vi "AlGaAs_seq_v00.vi"(2 "Debug Mode":bool, 3 "Elapsed Time(s)":dbl, 4 "State":enum16{"Edit", "Start", "Run", "End", "Idle"}(ring), 5 "Argument List In":string[](array[string])) -> (0 "Status Out":string, 1 "Argument List Out":string[](array[string]))   [LabVIEW 2011]
panel:
  out "time array":dbl[](array[numeric])
  out "nPeriod":dbl
  out "tTotal(s) 2":dbl
  out "is_OK":bool
  out "tSequence(s)":dbl
  in  "Tab Control":enum32{"Step 1", "Step 2", "Step 3", "Step 4"}(tab)
  in  "run Ga 1":bool caption="run Ga"
  in  "run Al 1":bool caption="run Al"
  in  "Al flow 1":dbl caption="Al flow(0-100sccm)" format="%.1f"
  in  "time 1":dbl caption="time(s)"
  in  "Ga flow 1":dbl caption="Ga flow(0-10sccm)" format="%.3f"
  in  "fGa dilution 1":dbl=1.0 caption="fGa dilution(>=1)"
  in  "run Ga 2":bool caption="run Ga"
  in  "run Al 2":bool caption="run Al"
  in  "fGa dilution 2":dbl=1.0 caption="fGa dilution(>=1)"
  in  "Al flow 2":dbl caption="Al flow (0-100sccm)" format="%.1f"
  in  "Ga flow 2":dbl caption="Ga flow (0-10sccm)" format="%.3f"
  in  "time 2":dbl caption="time(s)"
  in  "time 3":dbl caption="time(s)"
  in  "Al flow 3":dbl caption="Al flow (0-100sccm)" format="%.1f"
  in  "run Al 3":bool caption="run Al"
  in  "Ga flow 3":dbl caption="Ga flow (0-10sccm)" format="%.3f"
  in  "fGa dilution 3":dbl=1.0 caption="fGa dilution(>=1)"
  in  "run Ga 3":bool caption="run Ga"
  in  "time 4":dbl caption="time(s)"
  in  "Al flow 4":dbl caption="Al flow (0-100sccm)" format="%.1f"
  in  "run Al 4":bool caption="run Al"
  in  "Ga flow 4":dbl caption="Ga flow (0-10sccm)" format="%.3f"
  in  "fGa dilution 4":dbl=1.0 caption="fGa dilution(>=1)"
  in  "run Ga 4":bool caption="run Ga"
  out "tphase(s)":dbl[](array[numeric])
  out "phase":i32
  in  "Cancel":bool
  in  "OK":bool
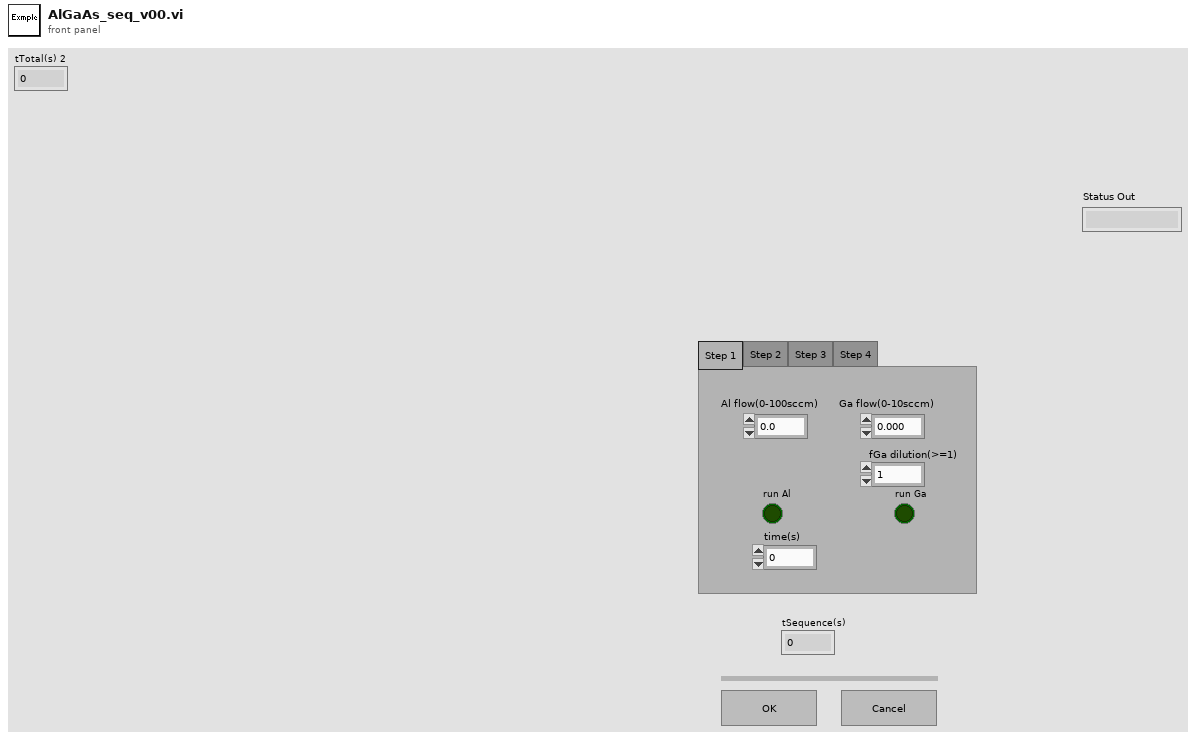
[diagram p1: front panel]
types:
  T1 = enum16{"Discrete", "Continuous", "Instantaneous"}
  T2 = enum32{"Invalid", "Default", "Floating", "Floating/Auto-Hide", "Modal"}
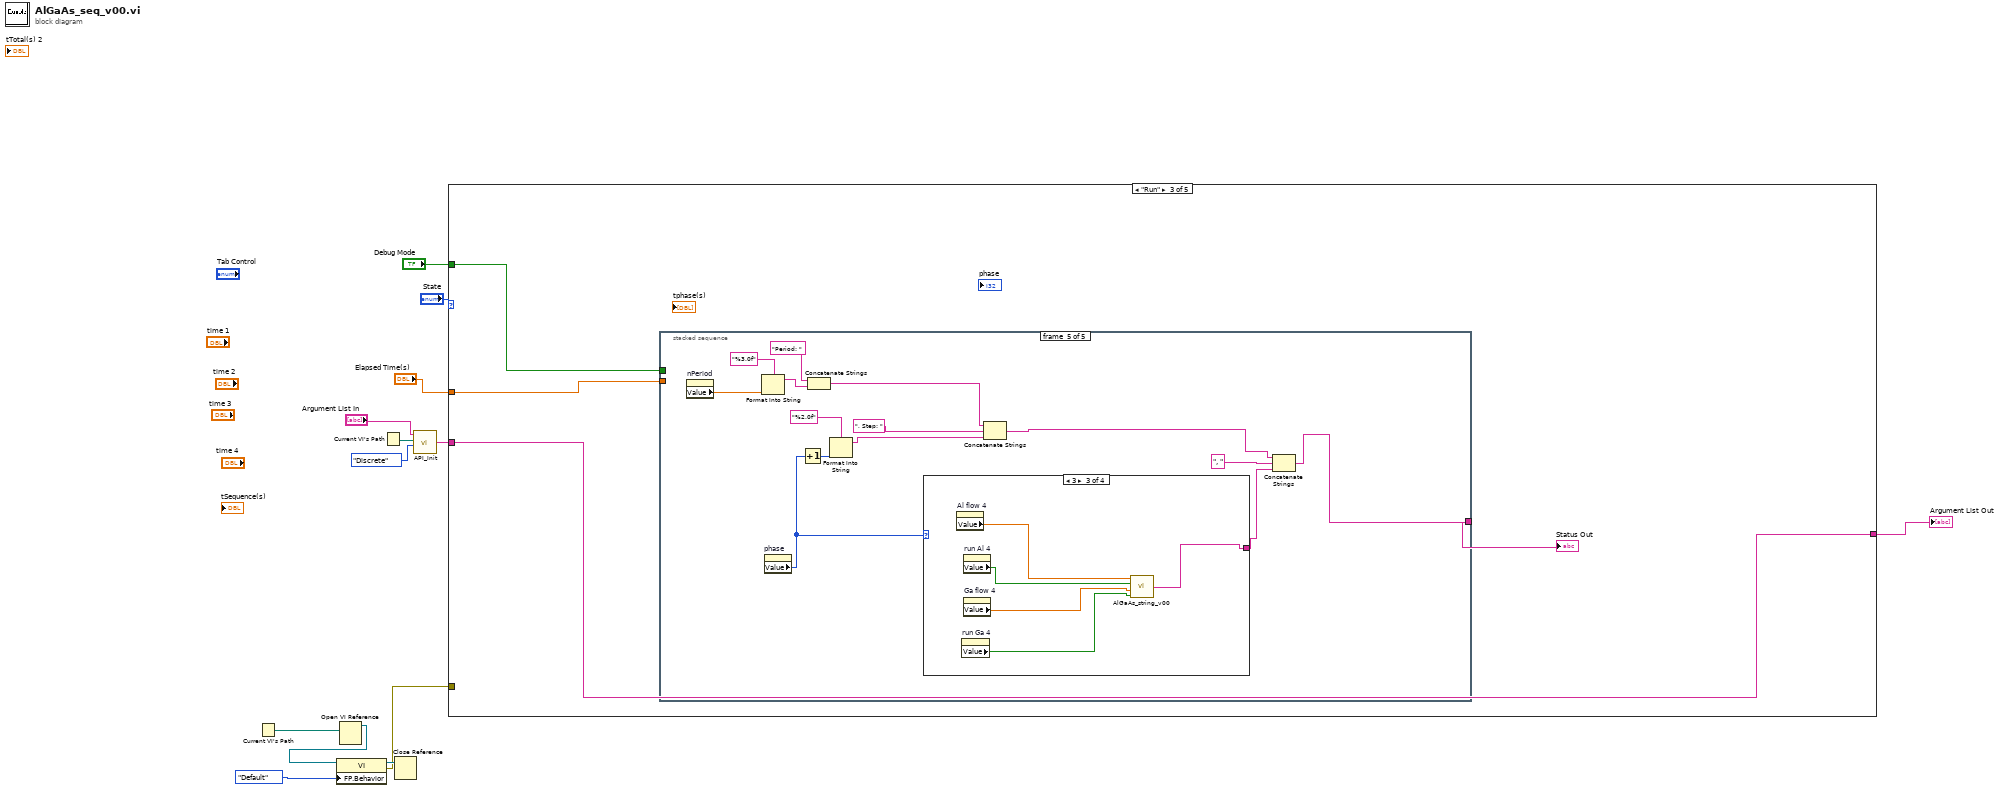
[diagram p0: block diagram]
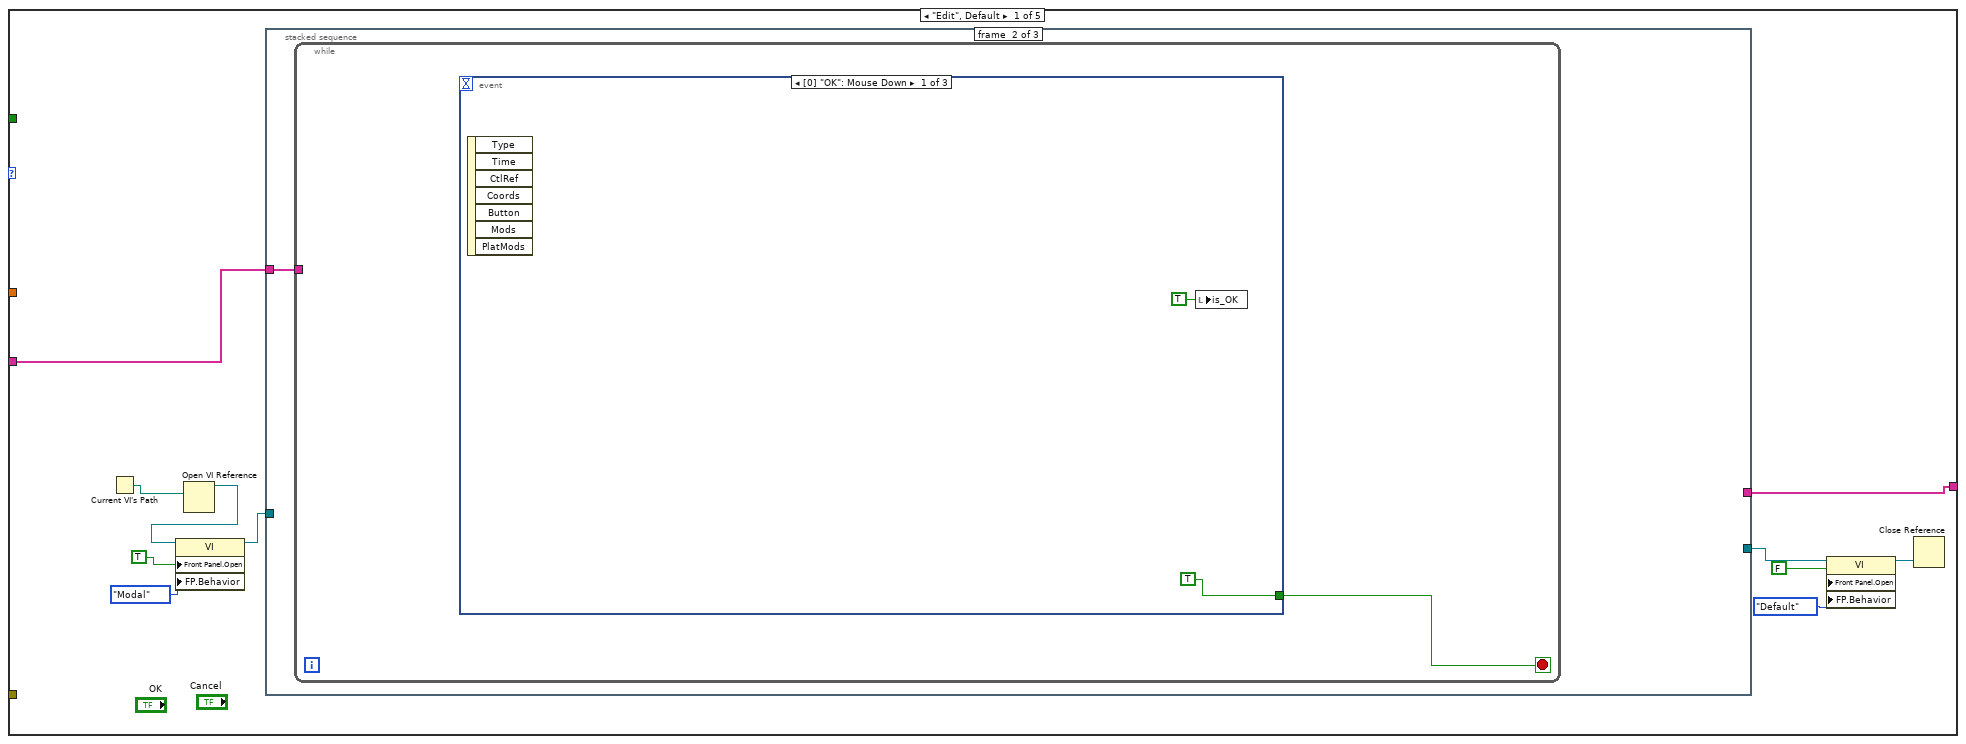
[diagram p2: hidden frame]
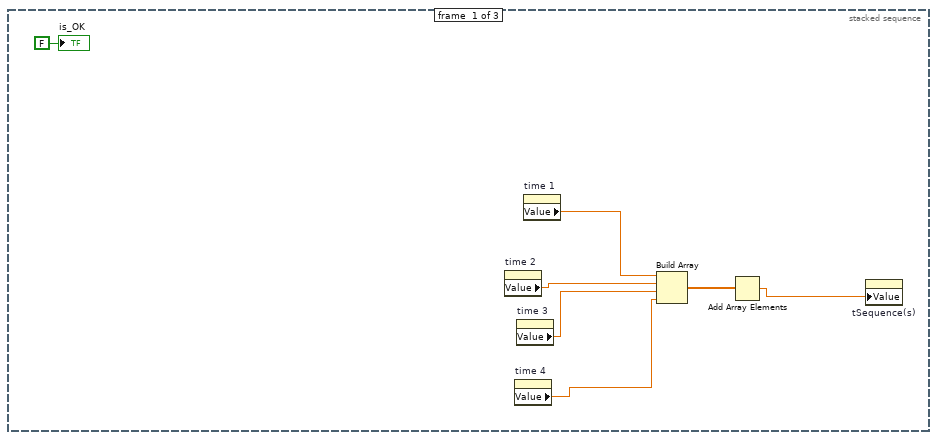
[diagram p3: hidden frame]
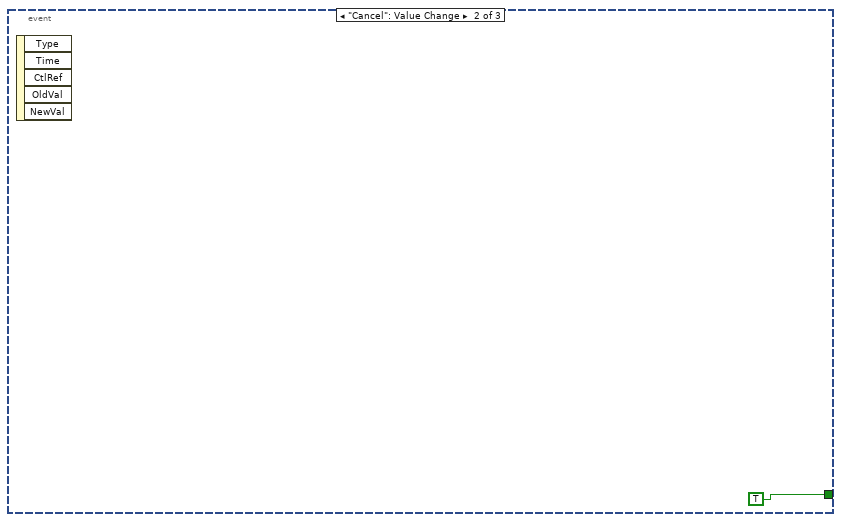
[diagram p4: hidden frame]
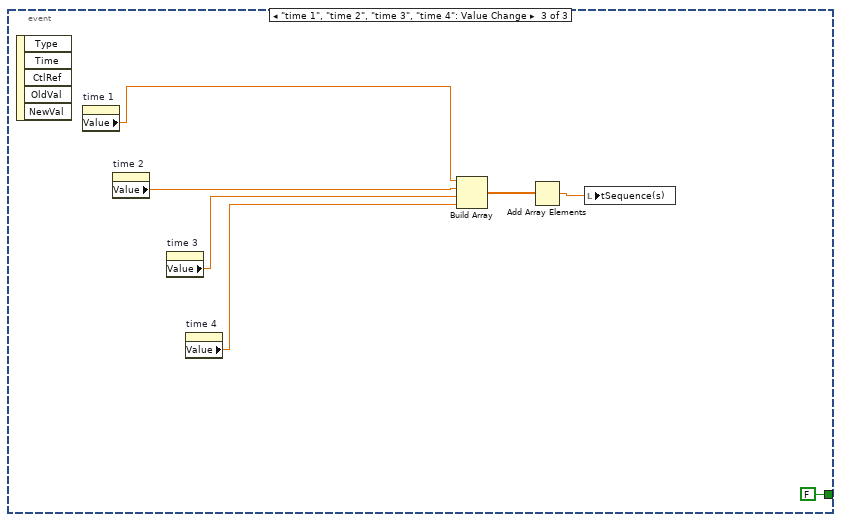
[diagram p5: hidden frame]
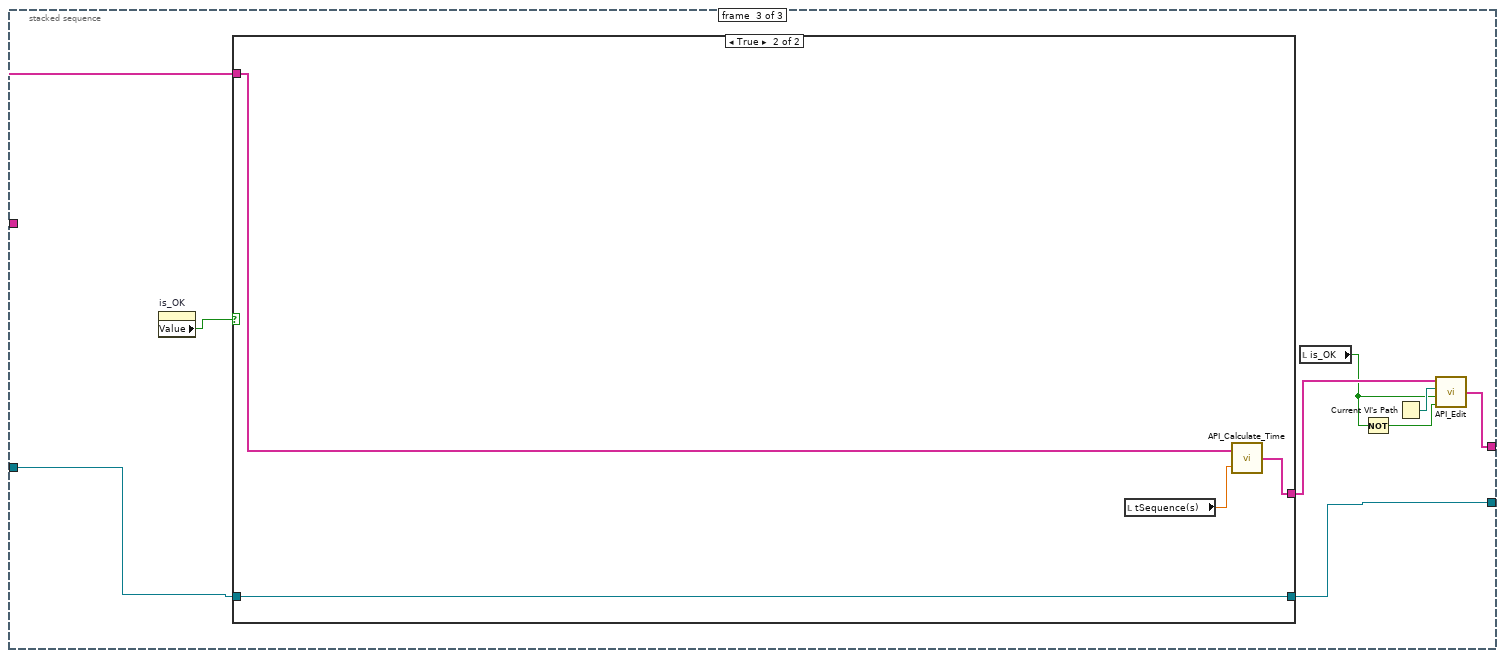
[diagram p6: hidden frame]
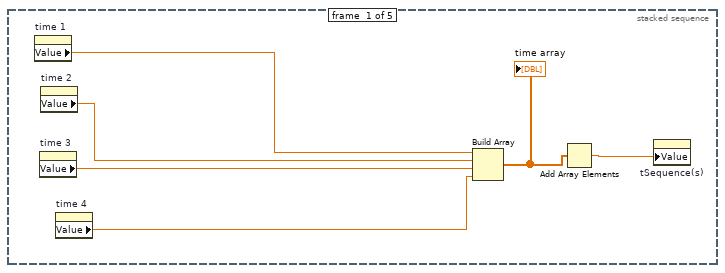
[diagram p9: hidden frame]
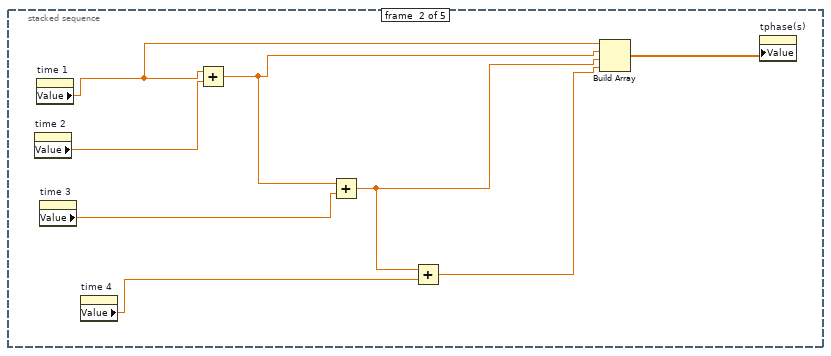
[diagram p10: hidden frame]
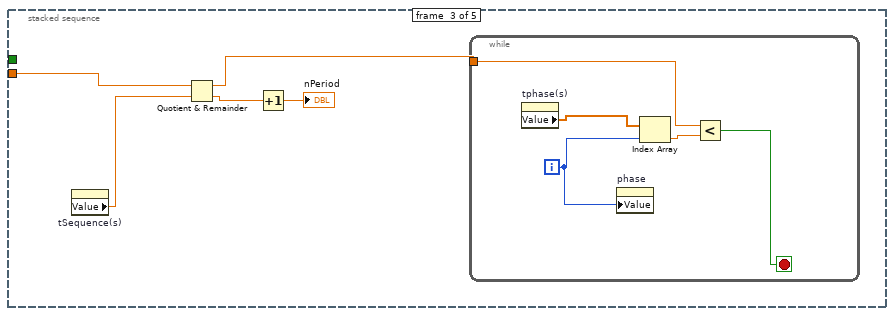
[diagram p11: hidden frame]
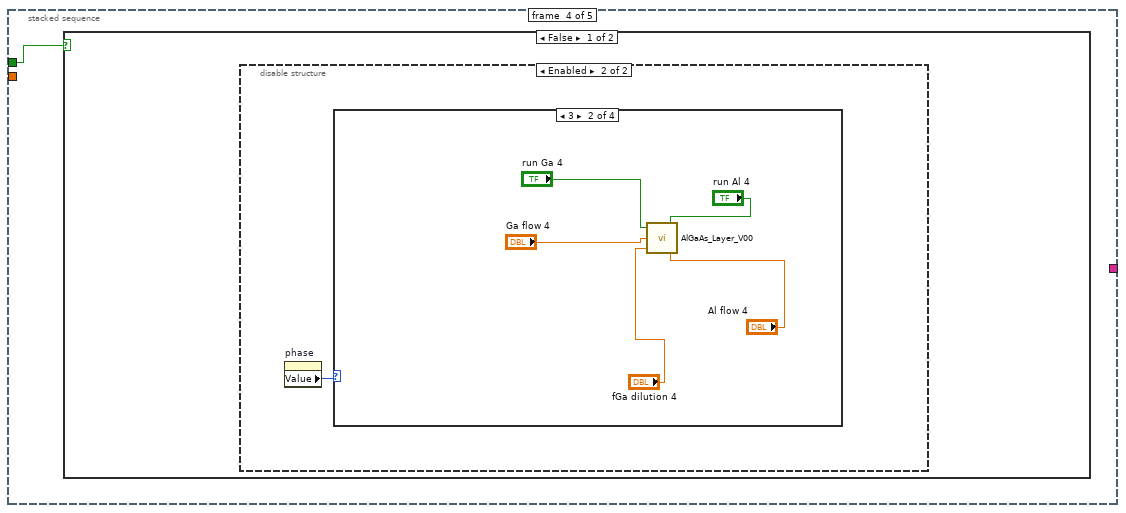
[diagram p12: hidden frame]
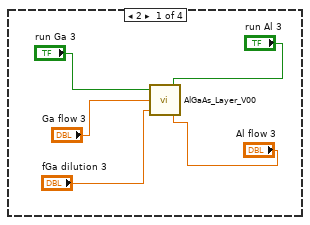
[diagram p14: hidden frame]
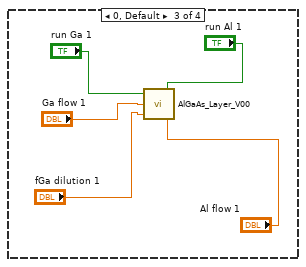
[diagram p15: hidden frame]
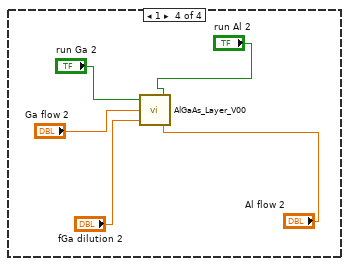
[diagram p16: hidden frame]
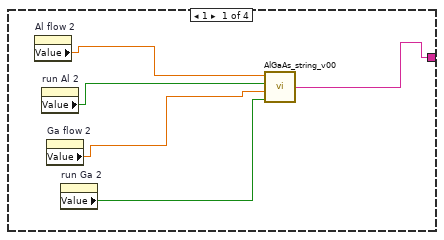
[diagram p18: hidden frame]
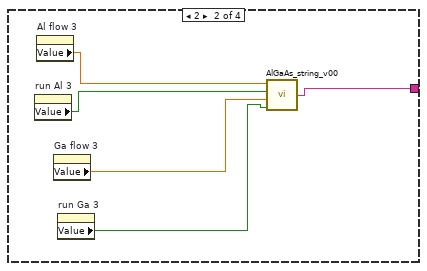
[diagram p19: hidden frame]
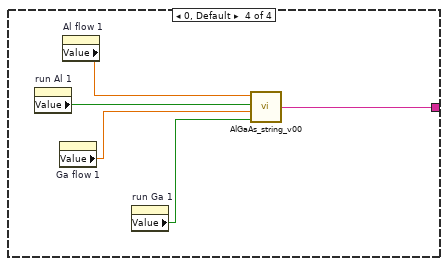
[diagram p20: hidden frame]
diagram:
  n1 = Current VI's Path() -> (path=w9:path)
  n2 = Open VI Reference(vi path=w9) -> (vi reference=w8:refnum<vi>)  [unwired: 1 in, 5 out]
  n3 = property class="VI"(reference=w8, "FP.Behavior"=T2."Default" ("Front Panel Window:Behavior")) -> (reference out=w6:refnum<vi>, error out=w5:errorcluster)  [unwired: 1 in]
  n4 = Current VI's Path() -> (path=w4:path)
  n5 = Close Reference(reference=w6) -> ()  [unwired: 1 in, 1 out]
  n6 = call "API_Init.vi"("API Mode"=T1."Discrete", "VI Path"=w4, "Argument List In"="Argument List In") -> ("Argument List Out"=w1:string[])  [unwired: 1 in]
  n7 = case shown="\"Run\"" "State" {
    tunnel: "Debug Mode" -> [_ _ w62 _ _]
    tunnel: "Elapsed Time(s)" -> [_ _ w63 _ _]
    tunnel: w1 -> [w14 w59 w60 w144 w145]
    tunnel: [w21 w59 w60 w144 w145] -> w10
    tunnel: w5 -> [_ _ _ _ _]
    frame "Edit", Default {
      n8 = Current VI's Path() -> (path=w19:path)
      n9 = Open VI Reference(vi path=w19) -> (vi reference=w18:refnum<vi>)  [unwired: 1 in, 5 out]
      n10 = property class="VI"(reference=w18, "Front Panel.Open"=TRUE ("Front Panel Window:Open"), "FP.Behavior"=T2."Modal" ("Front Panel Window:Behavior")) -> (reference out=w17:refnum<vi>)  [unwired: 1 in, 1 out]
      n11 = stacked-sequence {
        tunnel: w14 -> [_ w32 w52]
        tunnel: w17 -> [_ _ w50]
        tunnel: [_ _ w49] -> w22
        tunnel: [_ _ w46] -> w21
        frame #0 {
          n12 = property on="time 2" class="DigNum (strict)"() -> ("Value"=w27:dbl)  [unwired: 2 in, 2 out]
          n13 = property on="time 4" class="DigNum (strict)"() -> ("Value"=w25:dbl)  [unwired: 2 in, 2 out]
          n14 = property on="time 3" class="DigNum (strict)"() -> ("Value"=w26:dbl)  [unwired: 2 in, 2 out]
          n15 = property on="time 1" class="DigNum (strict)"() -> ("Value"=w30:dbl)  [unwired: 2 in, 2 out]
          n16 = Build Array(w30, w27, w26, w25) -> (w31:dbl[])
          n17 = Add Array Elements(numeric array=w31) -> (sum=w28:dbl)
          n18 = property on="tSequence(s)" class="DigNum (strict)"("Value"=w28) -> ()  [unwired: 2 in, 2 out]
          "is_OK" <- FALSE ("is_OK")
        }
        frame #1 {
          n19 = while {
            tunnel: w32 -> [_]
            stop <- w33 stop-if-true
            n20 = event shown="[0] \"OK\": Mouse Down" {
              selector: _ -> [_ _ _]
              dyn-events: _ -> [_ _ _]
              timeout: _ -> [_ _ _]
              tunnel: [TRUE ("done_editing") TRUE ("done_editing") FALSE ("done_editing")] -> w33
              event "OK": Mouse Down {
                n21 = event-data() -> ()  [unwired: 1 in, 7 out]
                n22 = local write "is_OK"(TRUE ("is_OK")) -> ()
              }
              event "Cancel": Value Change {
                n23 = event-data() -> ()  [unwired: 1 in, 5 out]
              }
              event "time 1", "time 2", "time 3", "time 4": Value Change {
                n24 = event-data() -> ()  [unwired: 1 in, 5 out]
                n25 = property on="time 1" class="DigNum (strict)"() -> ("Value"=w42:dbl)  [unwired: 2 in, 2 out]
                n26 = property on="time 2" class="DigNum (strict)"() -> ("Value"=w39:dbl)  [unwired: 2 in, 2 out]
                n27 = property on="time 3" class="DigNum (strict)"() -> ("Value"=w38:dbl)  [unwired: 2 in, 2 out]
                n28 = property on="time 4" class="DigNum (strict)"() -> ("Value"=w37:dbl)  [unwired: 2 in, 2 out]
                n29 = Build Array(w42, w39, w38, w37) -> (w41:dbl[])
                n30 = Add Array Elements(numeric array=w41) -> (sum=w40:dbl)
                n31 = local write "tSequence(s)"(w40) -> ()
              }
            }
          }
        }
        frame #2 {
          n32 = property on="is_OK" class="Bool (strict)"() -> ("Value"=w51:bool)  [unwired: 2 in, 2 out]
          n33 = case shown="True" w51 {
            tunnel: w52 -> [w54 w55]
            tunnel: [w54 w57] -> w47
            tunnel: w50 -> [w53 w58]
            tunnel: [w53 w58] -> w49
            frame False {
            }
            frame True {
              n34 = local read "tSequence(s)"() -> (w56:dbl)
              n35 = call "API_Calculate_Time.vi"("Time"=w56, "Argument List In"=w55) -> ("Argument List Out"=w57:string[])
            }
          }
          n36 = local read "is_OK"() -> (w45:bool)
          n37 = Not(x=w45) -> (.not. x?=w44:bool)
          n38 = Current VI's Path() -> (path=w48:path)
          n39 = call "API_Edit.vi"("Cancel"=w44, "OK"=w45, "VI Path"=w48, "Argument List In"=w47) -> ("Argument List Out"=w46:string[])
        }
      }
      n40 = property class="VI"(reference=w22, "Front Panel.Open"=FALSE ("Front Panel Window:Open"), "FP.Behavior"=T2."Default" ("Front Panel Window:Behavior")) -> (reference out=w23:refnum<vi>)  [unwired: 1 in, 1 out]
      n41 = Close Reference(reference=w23) -> ()  [unwired: 1 in, 1 out]
    }
    frame "Start" {
    }
    frame "Run" {
      n42 = stacked-sequence {
        tunnel: w63 -> [_ _ w82 _ _]
        tunnel: w62 -> [_ _ _ w88 _]
        tunnel: [_ _ _ _ w123] -> w61
        frame #0 {
          n43 = property on="time 1" class="DigNum (strict)"() -> ("Value"=w68:dbl)  [unwired: 2 in, 2 out]
          n44 = property on="time 3" class="DigNum (strict)"() -> ("Value"=w66:dbl)  [unwired: 2 in, 2 out]
          n45 = property on="time 2" class="DigNum (strict)"() -> ("Value"=w67:dbl)  [unwired: 2 in, 2 out]
          n46 = property on="time 4" class="DigNum (strict)"() -> ("Value"=w65:dbl)  [unwired: 2 in, 2 out]
          n47 = Build Array(w68, w67, w66, w65) -> (w64:dbl[])
          "time array" <- w64
          n48 = Add Array Elements(numeric array=w64) -> (sum=w69:dbl)
          n49 = property on="tSequence(s)" class="DigNum (strict)"("Value"=w69) -> ()  [unwired: 2 in, 2 out]
        }
        frame #1 {
          n50 = property on="time 2" class="DigNum (strict)"() -> ("Value"=w75:dbl)  [unwired: 2 in, 2 out]
          n51 = property on="time 1" class="DigNum (strict)"() -> ("Value"=w76:dbl)  [unwired: 2 in, 2 out]
          n52 = property on="time 3" class="DigNum (strict)"() -> ("Value"=w73:dbl)  [unwired: 2 in, 2 out]
          n53 = property on="time 4" class="DigNum (strict)"() -> ("Value"=w71:dbl)  [unwired: 2 in, 2 out]
          n54 = Add(x=w76, y=w75) -> (x+y=w74:dbl)
          n55 = Add(x=w74, y=w73) -> (x+y=w72:dbl)
          n56 = Add(x=w72, y=w71) -> (x+y=w70:dbl)
          n57 = Build Array(w76, w74, w72, w70) -> (w77:dbl[])
          n58 = property on="tphase(s)" class="Arr (strict)"("Value"=w77) -> ()  [unwired: 2 in, 2 out]
        }
        frame #2 {
          n59 = property on="tSequence(s)" class="DigNum (strict)"() -> ("Value"=w80:dbl)  [unwired: 2 in, 2 out]
          n60 = Quotient & Remainder(x=w82, y=w80) -> (x-y*floor(x/y)=w81:dbl, floor(x/y)=w79:dbl)
          n61 = Increment(x=w79) -> (x+1=→"nPeriod":dbl)
          n62 = while {
            tunnel: w81 -> [w86]
            i -> [w84]
            stop <- w83 stop-if-true
            n63 = property on="tphase(s)" class="Arr (strict)"() -> ("Value"=w87:dbl[])  [unwired: 2 in, 2 out]
            n64 = property on="phase" class="DigNum (strict)"("Value"=w84) -> ()  [unwired: 2 in, 2 out]
            n65 = Index Array(array=w87, index=w84) -> (element=w85:dbl)
            n66 = Less?(x=w86, y=w85) -> (x < y?=w83:bool)
          }
        }
        frame #3 {
          n67 = case shown="False" w88 {
            frame False {
              n68 = disable-structure shown="Enabled" {
                frame Disabled {
                }
                frame Enabled {
                  n69 = property on="phase" class="DigNum (strict)"() -> ("Value"=w89:i32)  [unwired: 2 in, 2 out]
                  n70 = case shown="3" w89 {
                    frame 2 {
                      n71 = call "AlGaAs_Layer_V00.vi"("Aluminum Flow"="Al flow 3", "Al Run"="run Al 3", "fDilution"="fGa dilution 3", "Ga flow (0-10 sccm)"="Ga flow 3", "Ga Run"="run Ga 3") -> ()
                    }
                    frame 3 {
                      n72 = call "AlGaAs_Layer_V00.vi"("Aluminum Flow"="Al flow 4", "Al Run"="run Al 4", "fDilution"="fGa dilution 4", "Ga flow (0-10 sccm)"="Ga flow 4", "Ga Run"="run Ga 4") -> ()
                    }
                    frame 0, Default {
                      n73 = call "AlGaAs_Layer_V00.vi"("Aluminum Flow"="Al flow 1", "Al Run"="run Al 1", "fDilution"="fGa dilution 1", "Ga flow (0-10 sccm)"="Ga flow 1", "Ga Run"="run Ga 1") -> ()
                    }
                    frame 1 {
                      n74 = call "AlGaAs_Layer_V00.vi"("Aluminum Flow"="Al flow 2", "Al Run"="run Al 2", "fDilution"="fGa dilution 2", "Ga flow (0-10 sccm)"="Ga flow 2", "Ga Run"="run Ga 2") -> ()
                    }
                  }
                }
              }
            }
            frame True {
            }
          }
        }
        frame #4 {
          n75 = property on="nPeriod" class="DigNum (strict)"() -> ("Value"=w115:dbl)  [unwired: 2 in, 2 out]
          n76 = Format Into String(format string="%3.0f", w115) -> (resulting string=w114:string)  [unwired: 2 in, 1 out]
          n77 = property on="phase" class="DigNum (strict)"() -> ("Value"=w117:i32)  [unwired: 2 in, 2 out]
          n78 = Increment(x=w117) -> (x+1=w116:i32)
          n79 = Concatenate Strings("Period: " ("string"), w114) -> (w111:string)
          n80 = Format Into String(format string="%2.0f", w116) -> (resulting string=w121:string)  [unwired: 2 in, 1 out]
          n81 = case shown="3" w117 {
            tunnel: [w124 w129 w134 w143] -> w110
            frame 1 {
              n82 = property on="Al flow 2" class="DigNum (strict)"() -> ("Value"=w128:dbl)  [unwired: 2 in, 2 out]
              n83 = property on="run Al 2" class="Bool (strict)"() -> ("Value"=w127:bool)  [unwired: 2 in, 2 out]
              n84 = property on="Ga flow 2" class="DigNum (strict)"() -> ("Value"=w126:dbl)  [unwired: 2 in, 2 out]
              n85 = property on="run Ga 2" class="Bool (strict)"() -> ("Value"=w125:bool)  [unwired: 2 in, 2 out]
              n86 = call "AlGaAs_string_v00.vi"("Ga run"=w125, "RGa"=w126, "Al run"=w127, "RAl"=w128) -> ("result"=w124:string)
            }
            frame 2 {
              n87 = property on="run Al 3" class="Bool (strict)"() -> ("Value"=w132:bool)  [unwired: 2 in, 2 out]
              n88 = property on="Al flow 3" class="DigNum (strict)"() -> ("Value"=w133:dbl)  [unwired: 2 in, 2 out]
              n89 = property on="Ga flow 3" class="DigNum (strict)"() -> ("Value"=w131:dbl)  [unwired: 2 in, 2 out]
              n90 = property on="run Ga 3" class="Bool (strict)"() -> ("Value"=w130:bool)  [unwired: 2 in, 2 out]
              n91 = call "AlGaAs_string_v00.vi"("Ga run"=w130, "RGa"=w131, "Al run"=w132, "RAl"=w133) -> ("result"=w129:string)
            }
            frame 3 {
              n92 = property on="Al flow 4" class="DigNum (strict)"() -> ("Value"=w138:dbl)  [unwired: 2 in, 2 out]
              n93 = property on="run Ga 4" class="Bool (strict)"() -> ("Value"=w135:bool)  [unwired: 2 in, 2 out]
              n94 = property on="run Al 4" class="Bool (strict)"() -> ("Value"=w137:bool)  [unwired: 2 in, 2 out]
              n95 = property on="Ga flow 4" class="DigNum (strict)"() -> ("Value"=w136:dbl)  [unwired: 2 in, 2 out]
              n96 = call "AlGaAs_string_v00.vi"("Ga run"=w135, "RGa"=w136, "Al run"=w137, "RAl"=w138) -> ("result"=w134:string)
            }
            frame 0, Default {
              n97 = property on="run Al 1" class="Bool (strict)"() -> ("Value"=w140:bool)  [unwired: 2 in, 2 out]
              n98 = property on="Ga flow 1" class="DigNum (strict)"() -> ("Value"=w141:dbl)  [unwired: 2 in, 2 out]
              n99 = property on="Al flow 1" class="DigNum (strict)"() -> ("Value"=w142:dbl)  [unwired: 2 in, 2 out]
              n100 = property on="run Ga 1" class="Bool (strict)"() -> ("Value"=w139:bool)  [unwired: 2 in, 2 out]
              n101 = call "AlGaAs_string_v00.vi"("Ga run"=w139, "RGa"=w141, "Al run"=w140, "RAl"=w142) -> ("result"=w143:string)
            }
          }
          n102 = Concatenate Strings(w111, ", Step: " ("string"), w121) -> (w119:string)
          n103 = Concatenate Strings(w119, ", " ("string"), w110) -> (w123:string)
        }
      }
      "Status Out" <- w61
    }
    frame "End" {
    }
    frame "Idle" {
    }
  }
  "Argument List Out" <- w10
